vi "Moxom Run.vi"() -> ()   [LabVIEW 2011]
uses:
  <vilib>/Platform/TimedLoop/XDataNode/timing_clust.ctl
  <vilib>/Platform/TimedLoop/XDataNode/nitl_modes.ctl
  <vilib>/Platform/TimedLoop/XDataNode/wakeup.ctl
  <instrlib>/Hokuyo URG Series/Public/Initialize-Standard.vi
  <vilib>/Utility/inputDevices.llb/joystickAcquire.vi
  <vilib>/Utility/inputDevices.llb/closeJoystick.vi
  <vilib>/Instr/_visa.llb/VISA Configure Serial Port (Instr).vi
  <vilib>/Platform/TimedLoop/XDataNode/XDataNode.xnode
  <instrlib>/Hokuyo URG Series/Hokuyo URG Series.lvlib
  <vilib>/Platform/TimedLoop/XDataNode/XDNodeRunTimeDep.lvlib
panel:
  out "Motor control string":string
  out "Motor Remote":cluster{"Left Motor":dbl, "Right Motor":dbl}
  out "Motor Auto":cluster{"Left Motor":dbl, "Right Motor":dbl}
  out "Stop Robot":bool
  out "Turn Left":bool
  out "Turn Right":bool
  in  "Lidar Serial Port":refnum<visa-resource-name>="COM12"
  out "Kill Switch Enabled":bool
  in  "Motor Controller\nSerial Port":refnum<visa-resource-name>="COM10"
  out "Auto Enabled":bool
  in  "Auto":bool
  in  "stop":bool
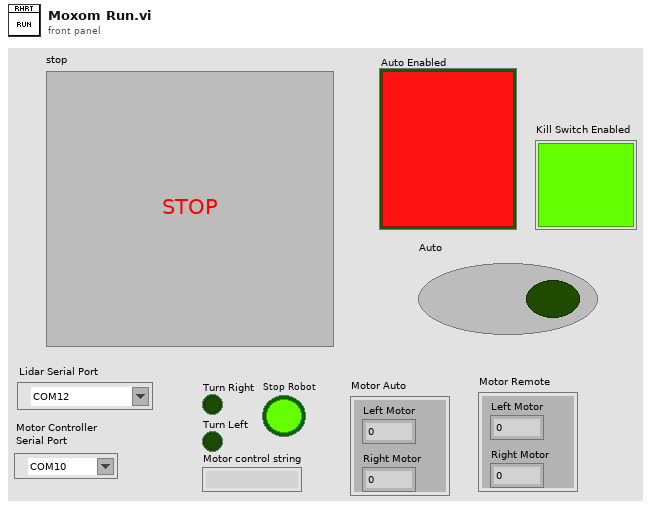
[diagram p1: front panel]
types:
  T1 = cluster{"axes total":u32, "buttons total":u32, "pov total":u32, "device name":string}[]
  T2 = cluster{"button 1":bool, "button 2":bool, "button 3":bool, "button 4":bool, "button 5":bool, "button 6":bool, "button 7":bool, "button 8":bool, "button 9":bool, "button 10":bool, "button 11":bool, "button 12":bool, "button 13":bool, "button 14":bool, "button 15":bool, "button 16":bool, "button 17":bool, "button 18":bool, "button 19":bool, "button 20":bool, "button 21":bool, "button 22":bool, "button 23":bool, "button 24":bool, "button 25":bool, "button 26":bool, "button 27":bool, "button 28":bool, "button 29":bool, "button 30":bool, "button 31":bool, "button 32":bool}
  T3 = typedef "XDNodeRunTimeDep.lvlib/timing_clust.ctl" = cluster{"Expected End [f-1]":u64, "Actual End [f-1]":u64, "Finished Late? [f-1]":bool, "Expected End [i-1]":u64, "Actual End [i-1]":u64, "Finished Late? [i-1]":bool, "Expected Start [i]":u64, "Actual Start [i]":u64, "Expected Start [f]":u64, "Actual Start [f]":u64, "Source Name":string, "Structure Name":string, "Period":i64, "Deadline":i64, "Offset":i64, "Start":i64, "Priority":i32, "Timeout":i32, "Mode":T4, "Wakeup Reason":T5, "Error":errorcluster, "Source Type":string, "Secondary Source Type":string, "Global End Time":u64, "Global Start Time":u64, "Frame Duration":u64, "Iteration Duration":u64, "Assigned CPU":i32, "I/O Scan Engine Mode":u32}
  T4 = typedef "XDNodeRunTimeDep.lvlib/nitl_modes.ctl" = enum32{"No Change", "Process missed periods, maintain original phase", "Discard missed periods, maintain original phase", "Process missed periods, ignore original phase", "Discard missed periods, ignore original phase"}
  T5 = typedef "XDNodeRunTimeDep.lvlib/wakeup.ctl" = enum32{"Normal", "Aborted", "Asynchronous wakeup", "Timing source error", "Timed loop error", "Timeout"}
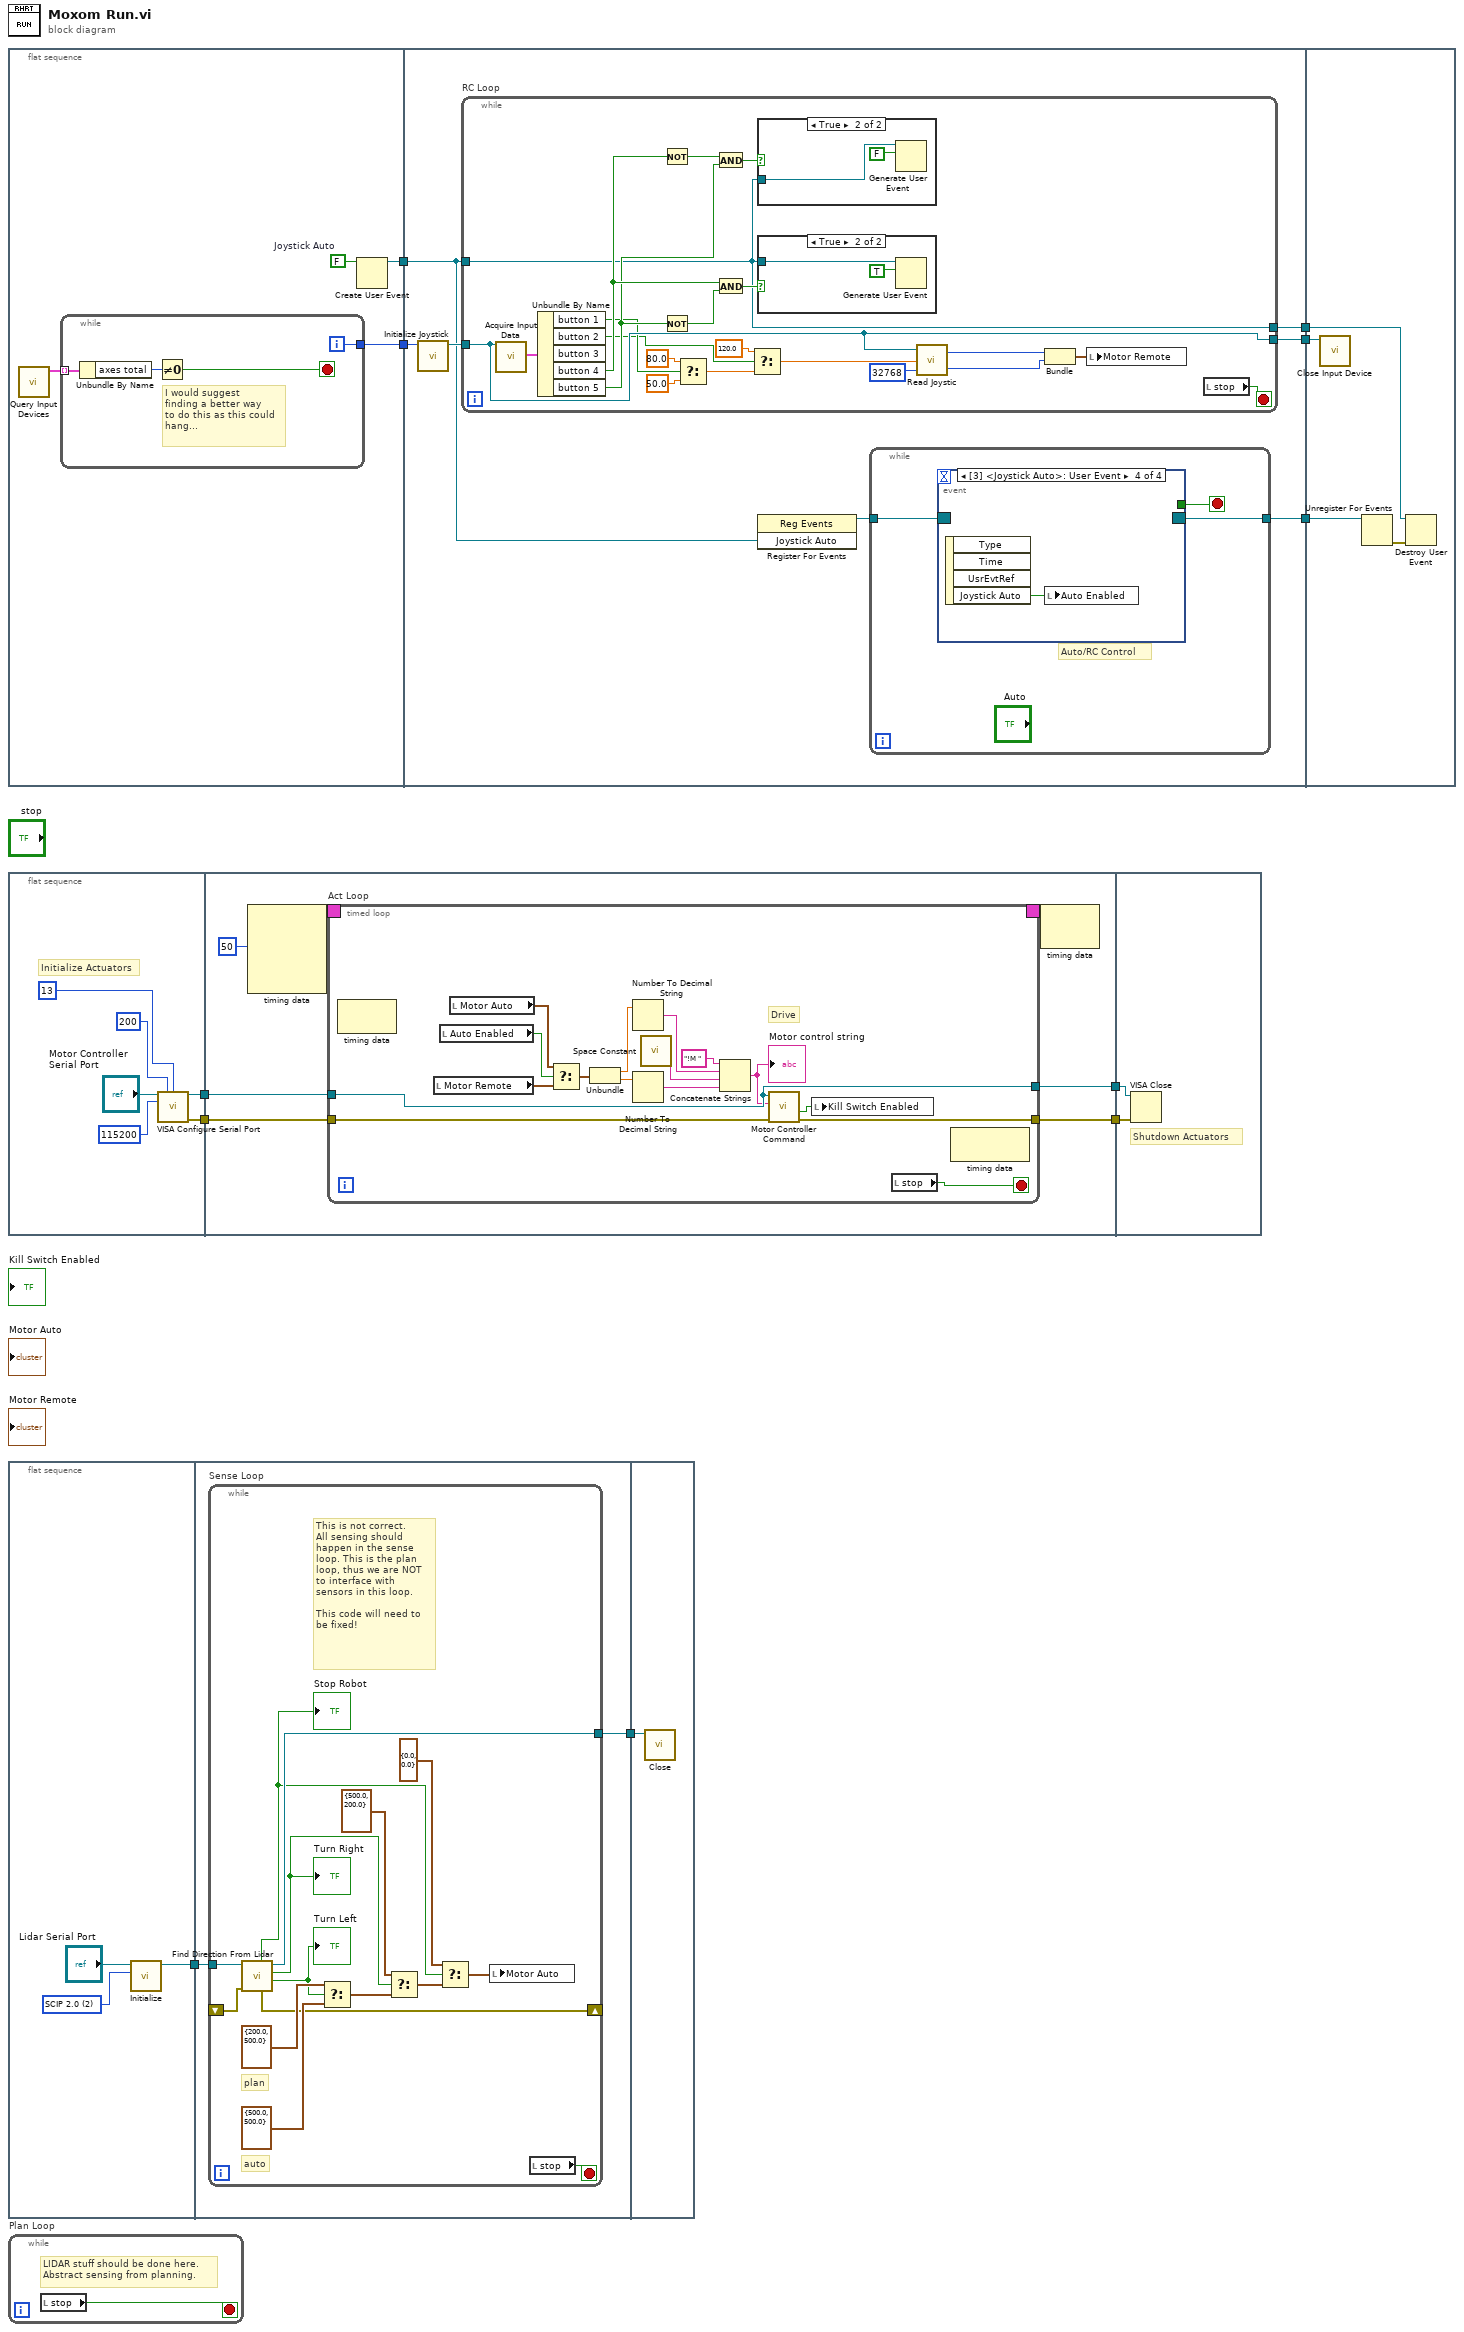
[diagram p0: block diagram]
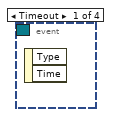
[diagram p4: hidden frame]
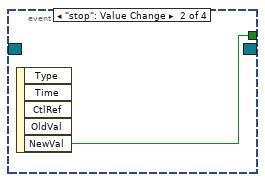
[diagram p5: hidden frame]
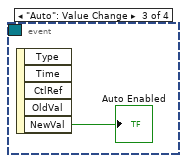
[diagram p6: hidden frame]
diagram:
  n1 = flat-sequence {
    tunnel: [w13] -> w6
    tunnel: [w12] -> w5
    tunnel: w6 -> [w24]
    tunnel: w5 -> [w23]
    tunnel: [w22] -> w4
    tunnel: [w21] -> w3
    tunnel: [w20] -> w2
    tunnel: w4 -> [w60]
    tunnel: w3 -> [w59]
    tunnel: w2 -> [w58]
    frame #0 {
      w14 = FALSE  # Joystick Auto
      n2 = call <vilib>:"Query Input Devices.vi"() -> ("joystick info"=w15:T1)  [unwired: 8 in, 3 out]
      n3 = while {
        tunnel: w15 -> [w19] mode=indexing
        tunnel: [w16] -> w12
        i -> [w16]
        stop <- w17 stop-if-true
        # "I would suggest\nfinding a better way\nto do this as this could\nhang..."
        n4 = Unbundle By Name(w19) -> ("axes total"=w18:u32)
        n5 = Not Equal To 0?(x=w18) -> (x != 0?=w17:bool)
      }
      n6 = Create User Event(user event datatype=w14) -> (user event=w13:refnum<user-event>)  [unwired: 1 in, 1 out]
    }
    frame #1 {
      n7 = call <vilib>:"Initialize Joystick.vi"("device index"=w23) -> ("device ID"=w25:refnum<k1>)  [unwired: 9 in, 1 out]
      n8 = while "RC Loop" {
        tunnel: w25 -> [w41]
        tunnel: [w41] -> w20
        tunnel: w24 -> [w34]
        tunnel: [w34] -> w22
        stop <- w47 stop-if-true
        n9 = call-poly <vilib>:"Acquire Input Data.vi"("device ID"=w41) -> ("button info"=w42:T2)  [unwired: 14 in, 4 out]
        n10 = Unbundle By Name(w42) -> ("button 1"=w33:bool, "button 2"=w27:bool, "button 4"=w38:bool, "button 5"=w37:bool)  [unwired: 1 out]
        n11 = Not(x=w38) -> (.not. x?=w36:bool)
        n12 = Not(x=w37) -> (.not. x?=w35:bool)
        n13 = Select(t=80.0, s=w33, f=50.0) -> (s? t:f=w30:dbl)
        n14 = And(x=w36, y=w37) -> (x .and. y?=w40:bool)
        n15 = And(x=w38, y=w35) -> (x .and. y?=w39:bool)
        n16 = Select(t=120.0, s=w27, f=w30) -> (s? t:f=w29:dbl)
        n17 = case shown="True" w40 {
          tunnel: w34 -> [_ w48]
          frame False {
          }
          frame True {
            n18 = Generate User Event(user event=w48, event data cluster=FALSE ("Auto Enabled")) -> ()  [unwired: 1 in, 2 out]
          }
        }
        n19 = case shown="True" w39 {
          tunnel: w34 -> [_ w50]
          frame False {
          }
          frame True {
            n20 = Generate User Event(user event=w50, event data cluster=TRUE ("Auto Enabled")) -> ()  [unwired: 1 in, 2 out]
          }
        }
        n21 = call "Read Joystic.vi"("JoystickOutMaximum"=32768, "MaxMotorSpeed"=w29, "device ID"=w41) -> ("Right Motor"=w43:i32, "Left Motor"=w44:i32)
        n22 = Bundle("Left Motor"=w44, "Right Motor"=w43) -> (w45:cluster{"Left Motor":i32, "Right Motor":i32})  [unwired: 1 in]
        n23 = local write "Motor Remote"(w45) -> ()
        n24 = local read "stop"() -> (w47:bool)
      }
      n25 = register-events(w24) -> (reference out=w26:refnum<event-registration>)  [unwired: 2 in, 1 out]
      n26 = while {
        tunnel: w26 -> [w53]
        tunnel: [w52] -> w21
        stop <- w54 stop-if-true
        # "Auto/RC Control"
        n27 = event shown="[3] <Joystick Auto>: User Event" {
          selector: w53 -> [_ _ _ _]
          dyn-events: [_ _ _ _] -> w52
          timeout: _ -> [_ _ _ _]
          tunnel: [_ w55 _ _] -> w54
          event Timeout {
            n28 = event-data() -> ()  [unwired: 1 in, 2 out]
          }
          event "stop": Value Change {
            n29 = event-data() -> ("NewVal"=w55:bool)  [unwired: 1 in, 4 out]
          }
          event "Auto": Value Change {
            n30 = event-data() -> ("NewVal"=→"Auto Enabled":bool)  [unwired: 1 in, 4 out]
          }
          event User Event {
            n31 = event-data() -> ("Joystick Auto"=w57:bool)  [unwired: 1 in, 3 out]
            n32 = local write "Auto Enabled"(w57) -> ()
          }
        }
      }
    }
    frame #2 {
      n33 = call-poly <vilib>:"Close Input Device.vi"("device ID"=w58) -> ()  [unwired: 9 in, 1 out]
      n34 = Unregister For Events(event registration refnum=w59) -> (error out=w61:errorcluster)  [unwired: 1 in]
      n35 = Destroy User Event(user event=w60, error in=w61) -> ()  [unwired: 1 out]
    }
  }
  n36 = flat-sequence {
    tunnel: [w63] -> w10
    tunnel: [w62] -> w7
    tunnel: [w73] -> w11
    tunnel: w10 -> [w74]
    tunnel: [w72] -> w8
    tunnel: w7 -> [w71]
    tunnel: w11 -> [w98]
    tunnel: w8 -> [w97]
    frame #0 {
      # "Initialize Actuators"
      n37 = call-poly "VISA Configure Serial Port"("VISA resource name"="Motor Controller\nSerial Port", "timeout (10sec)"=u32 200, "termination char\n(0xA = '\\n' = LF)"=u8 13 ("termination char\n(0xA = '\\n' = LF)"), "baud rate (9600)"=u32 115200) -> ("VISA resource name out"=w63:refnum<visa-resource-name>, "error out"=w62:errorcluster)  [unwired: 10 in]
    }
    frame #1 {
      n38 = node-c288(i64 50 ("Period")) -> (w70:T3)  [unwired: 3 in]
      n39 = timed-loop "Act Loop" {
        tunnel: w74 -> [w86]
        tunnel: [w86] -> w73
        tunnel: [w76] -> w72
        tunnel: w71 -> [w75]
        timing: w70 -> [_]
        timing-out: [_] -> w69
        stop <- w90 stop-if-true
        # "Drive"
        n40 = node-c288() -> ()  [unwired: 1 in, 1 out]
        n41 = local read "Motor Remote"() -> (w81:cluster{"Left Motor":dbl, "Right Motor":dbl})
        n42 = local read "Auto Enabled"() -> (w89:bool)
        n43 = local read "Motor Auto"() -> (w80:cluster{"Left Motor":dbl, "Right Motor":dbl})
        n44 = Select(t=w80, s=w89, f=w81) -> (s? t:f=w79:cluster{"Left Motor":dbl, "Right Motor":dbl})
        n45 = Unbundle(w79) -> ("Left Motor"=w78:dbl, "Right Motor"=w77:dbl)
        n46 = Number To Decimal String(number=w78) -> (decimal integer string=w84:string)  [unwired: 1 in]
        n47 = Number To Decimal String(number=w77) -> (decimal integer string=w83:string)  [unwired: 1 in]
        n48 = call <vilib>:"Space Constant.vi"() -> ("String"=w87:string)
        n49 = Concatenate Strings("!M " ("string"), w84, w87, w83) -> (w85:string)
        "Motor control string" <- w85
        n50 = call "Motor Controller Command.vi"("error in (no error)"=w75, "Command"=w85, "VISA resource name"=w86) -> ("error out"=w76:errorcluster, "Timeout on read"=w82:bool)  [unwired: 5 in, 2 out]
        n51 = local write "Kill Switch Enabled"(w82) -> ()
        n52 = local read "stop"() -> (w90:bool)
        n53 = node-c288() -> ()  [unwired: 1 in, 1 out]
      }
      n54 = node-c288(w69) -> ()  [unwired: 1 out]
    }
    frame #2 {
      # "Shutdown Actuators"
      n55 = VISA Close(VISA resource name=w98, error in (no error)=w97) -> ()  [unwired: 1 out]
    }
  }
  n56 = flat-sequence {
    tunnel: [w99] -> w1
    tunnel: [w103] -> w9
    tunnel: w1 -> [w102]
    tunnel: w9 -> [w119]
    frame #0 {
      w101 = u32 2 items=["Convert to Latest", "SCIP 1.1", "SCIP 2.0"] ("Protocol (2: SCIP 2.0)")
      n57 = call-poly <instrlib>:"Initialize.vi"("Protocol (2: SCIP 2.0)"=w101, "VISA resource name"="Lidar Serial Port") -> ("VISA resource name out"=w99:refnum<visa-resource-name>)  [unwired: 8 in, 1 out]
    }
    frame #1 {
      n58 = while "Sense Loop" {
        shift-right: [w110] -> _
        shift-left: _ -> [w104]
        tunnel: [w109] -> w103
        tunnel: w102 -> [w105]
        stop <- w118 stop-if-true
        # "This is not correct. \nAll sensing should\nhappen in the sense\nloop. This is the plan\nloop, thus we are NOT\nto interface with \nsensors in this loop.\n\nThis code will need to\nbe fixed!"
        # "auto"
        # "plan"
        n59 = call "Find Direction From Lidar.vi"("error in (no error)"=w104, "VISA resource name"=w105) -> ("Turn Left"=w106:bool, "Turn Right"=w107:bool, "VISA resource name out"=w109:refnum<visa-resource-name>, "error out"=w110:errorcluster, "Stop Robot"=w108:bool)  [unwired: 4 in, 1 out]
        "Turn Right" <- w107
        "Turn Left" <- w106
        "Stop Robot" <- w108
        n60 = Select(t=cluster{"Left Motor":dbl, "Right Motor":dbl} {"Left Motor"=200.0, "Right Motor"=500.0} ("Motor Remote"), s=w106, f=cluster{"Left Motor":dbl, "Right Motor":dbl} {"Left Motor"=500.0, "Right Motor"=500.0} ("Motor Remote")) -> (s? t:f=w114:cluster{"Left Motor":dbl, "Right Motor":dbl})
        n61 = Select(t=cluster{"Left Motor":dbl, "Right Motor":dbl} {"Left Motor"=500.0, "Right Motor"=200.0} ("Motor Remote"), s=w107, f=w114) -> (s? t:f=w115:cluster{"Left Motor":dbl, "Right Motor":dbl})
        n62 = Select(t=cluster{"Left Motor":dbl, "Right Motor":dbl} {"Left Motor"=0.0, "Right Motor"=0.0} ("Motor Remote"), s=w108, f=w115) -> (s? t:f=w117:cluster{"Left Motor":dbl, "Right Motor":dbl})
        n63 = local write "Motor Auto"(w117) -> ()
        n64 = local read "stop"() -> (w118:bool)
      }
    }
    frame #2 {
      n65 = call <instrlib>:"Close.vi"("VISA resource name"=w119) -> ()  [unwired: 10 in, 1 out]
    }
  }
  n66 = while "Plan Loop" {
    stop <- w120 stop-if-true
    # "LIDAR stuff should be done here.\nAbstract sensing from planning."
    n67 = local read "stop"() -> (w120:bool)
  }
